vi "WPI_UtilitiesFRC ReadUserButton.vi"(8 "error in":errorcluster) -> (0 "error out":errorcluster, 3 "User Button":bool)   [LabVIEW 2019]
doc: "Returns the Boolean value of the USER button on the roboRIO. The value is True when the button is pressed.\n\nThis software is licensed. Open the labview\\readme\\WPI Robotics Library Open Source License.txt file for more information."
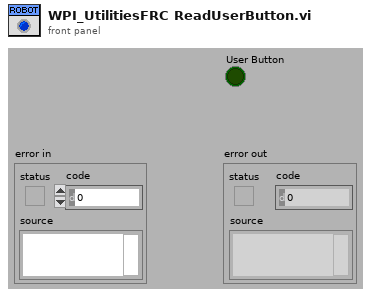
[diagram p1: front panel]
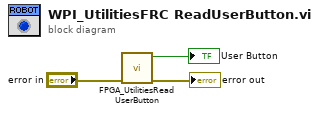
[diagram p0: block diagram]
diagram:
  n1 = call <vilib>:"FPGA_UtilitiesRead UserButton.vi"("error in (no error)"="error in") -> ("error out"=→"error out":errorcluster, "UserButton"=→"User Button":bool)  [unwired: 9 in]
